vi "EX_1_Llenado tanque máquina de esatados.vi"() -> ()   [LabVIEW 2026]
panel:
  out "MOTOR":bool
  out "V1":bool
  out "V2":bool
  out "VB":bool
  out "TANQUE VB":dbl(slide) scale=0.0..10.0
  out "TANQUE VA":dbl(slide) scale=0.0..10.0
  out "VA":bool
  out "TANQUE 1":dbl(slide) scale=0.0..20.0
  out "TANQUE 2":dbl(slide) scale=0.0..20.0
  in  "Inicio":bool
  in  "DL2":bool
  in  "DL1":bool
  in  "stop":bool
  in  "SP1":bool
  in  "SP2":bool
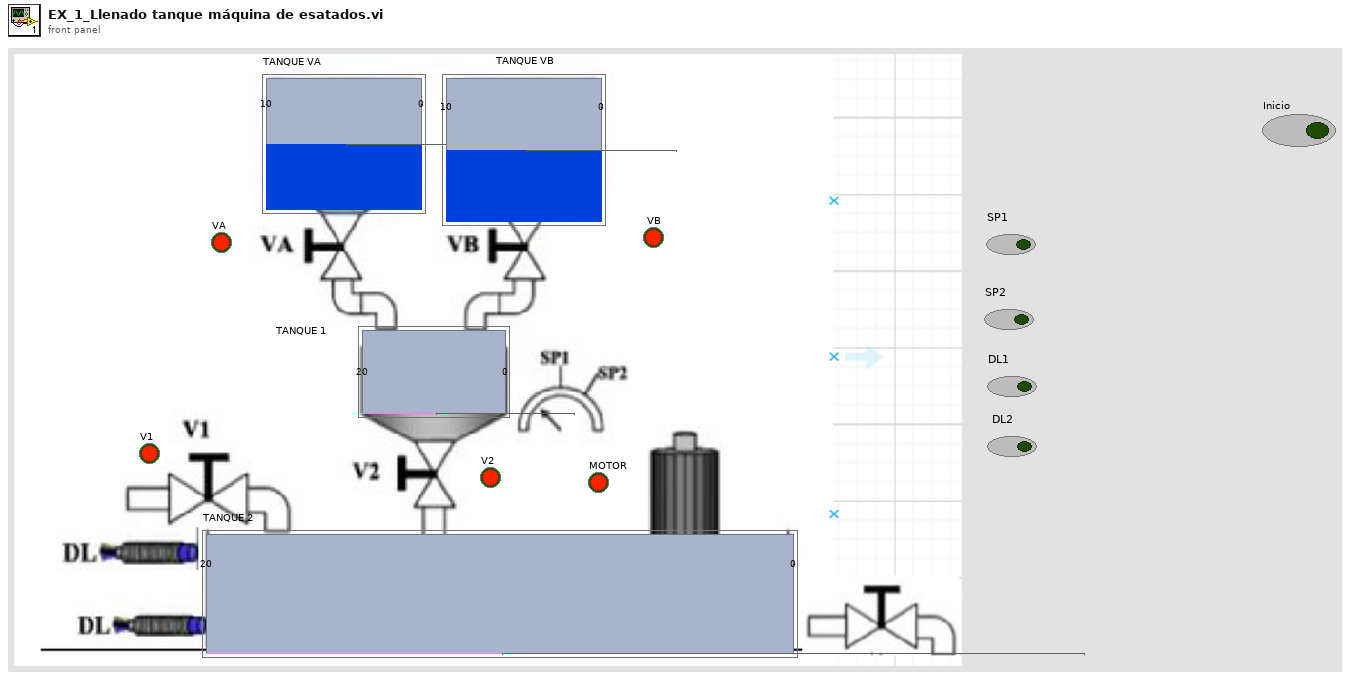
[diagram p1: front panel]
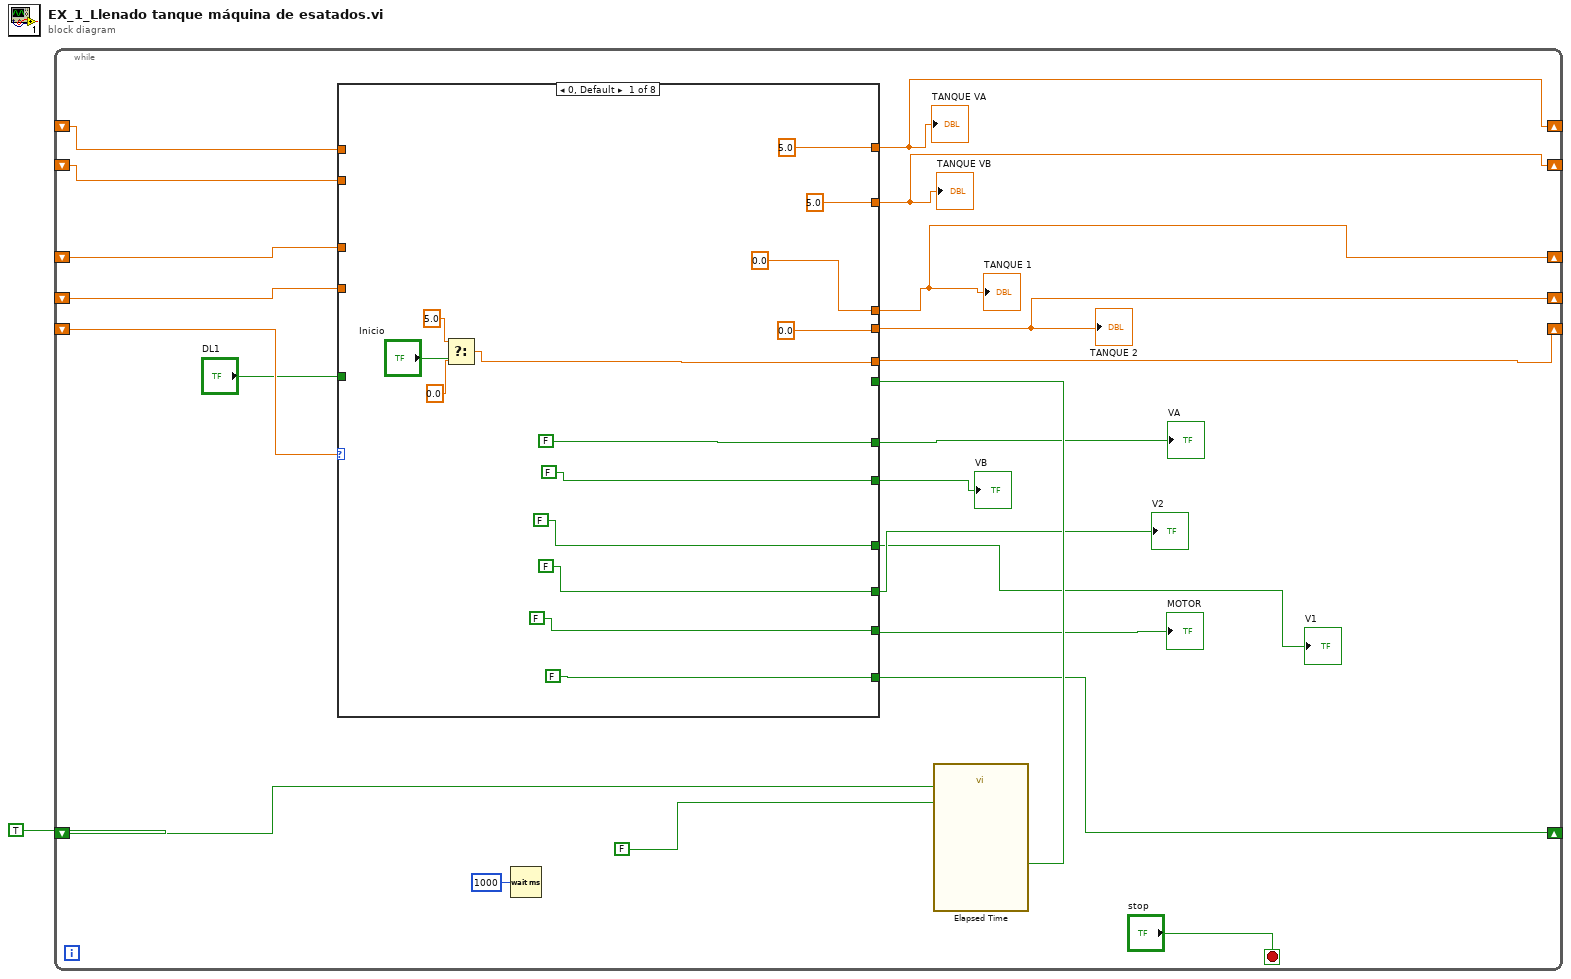
[diagram p0: block diagram]
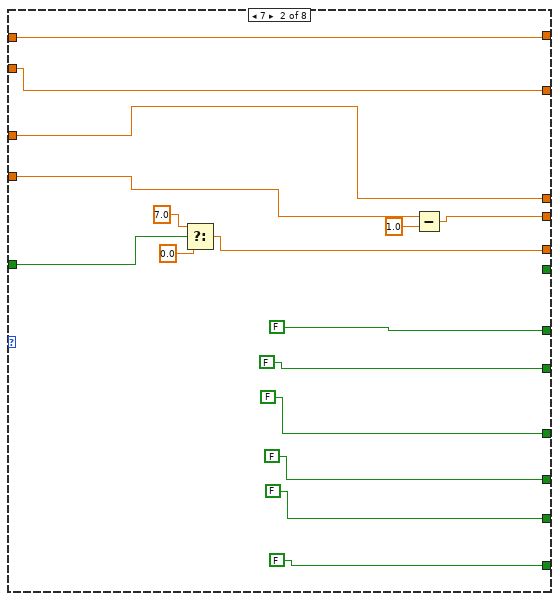
[diagram p2: hidden frame]
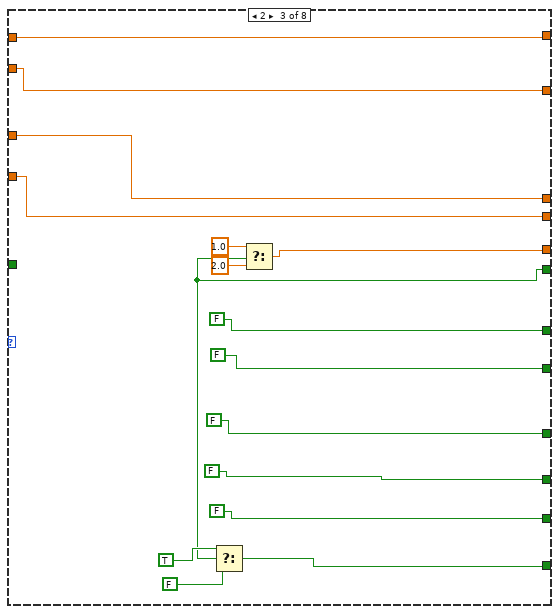
[diagram p3: hidden frame]
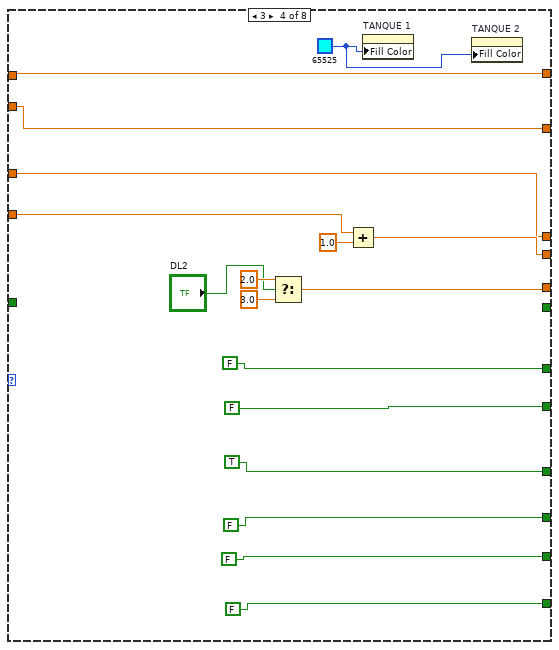
[diagram p4: hidden frame]
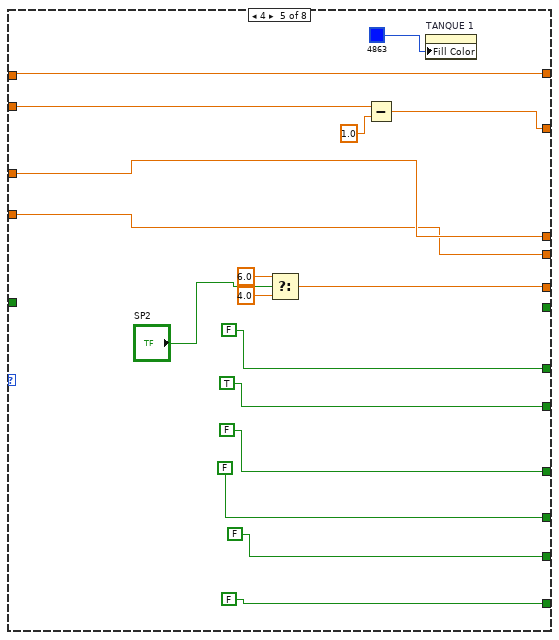
[diagram p5: hidden frame]
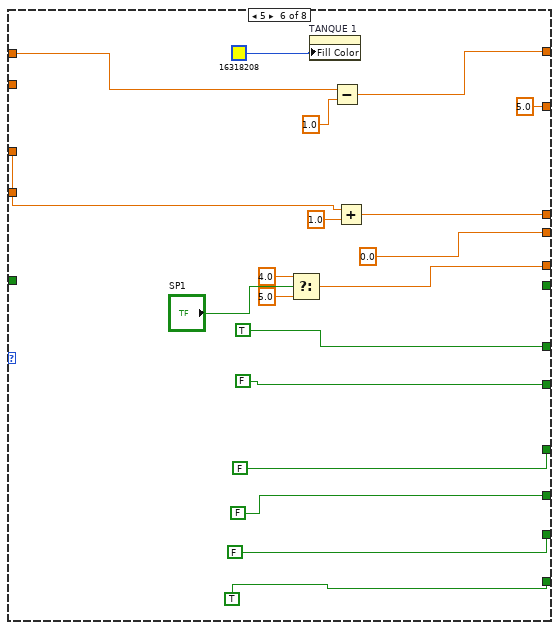
[diagram p6: hidden frame]
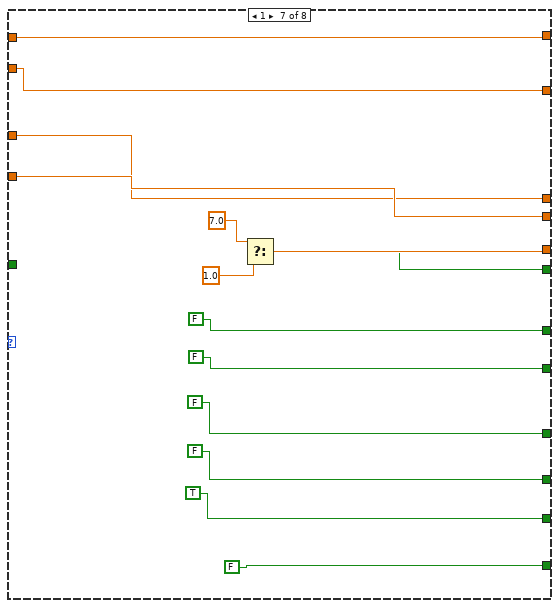
[diagram p7: hidden frame]
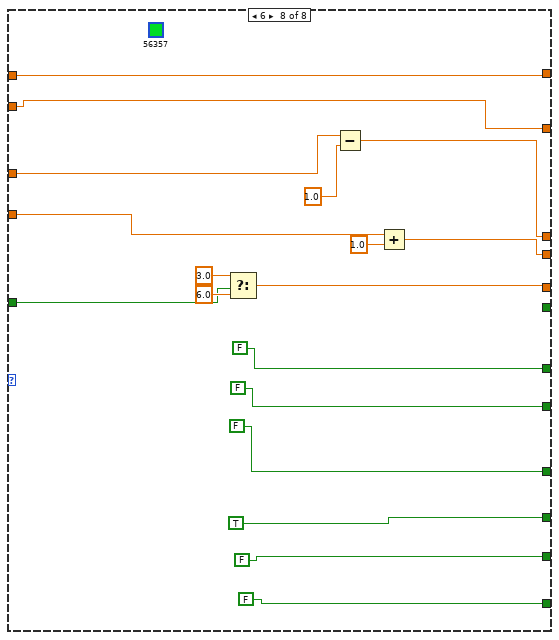
[diagram p8: hidden frame]
diagram:
  n1 = while {
    shift-right: [w21] -> _
    shift-left: _ -> [w23]
    shift-right: [w17] -> _
    shift-left: TRUE -> [w20]
    shift-right: [w13] -> _
    shift-left: _ -> [w14]
    shift-right: [w11] -> _
    shift-left: _ -> [w12]
    shift-right: [w9] -> _
    shift-left: _ -> [w7]
    shift-right: [w8] -> _
    shift-left: _ -> [w5]
    stop <- "stop" stop-if-true
    n2 = Wait (ms)(milliseconds to wait=u32 1000) -> ()  [unwired: 1 out]
    n3 = call "Elapsed Time"("Reset"=w20, "Auto Reset"=FALSE) -> ("Time has Elapsed"=w18:bool)  [unwired: 10 in, 7 out]
    n4 = case shown="0, Default" w23 {
      tunnel: [FALSE FALSE FALSE FALSE FALSE TRUE FALSE FALSE] -> w10
      tunnel: [FALSE FALSE FALSE FALSE TRUE FALSE FALSE FALSE] -> w4
      tunnel: [FALSE FALSE FALSE TRUE FALSE FALSE FALSE FALSE] -> w2
      tunnel: [FALSE FALSE FALSE FALSE FALSE FALSE FALSE TRUE] -> w3
      tunnel: [FALSE FALSE FALSE FALSE FALSE FALSE TRUE FALSE] -> w6
      tunnel: [w30 w53 w64 w81 w96 w116 w129 w150] -> w21
      tunnel: w18 -> [_ _ w58 _ _ _ w128 _]
      tunnel: [FALSE FALSE w59 FALSE FALSE TRUE FALSE FALSE] -> w17
      tunnel: [0.0 w41 w54 w73 w91 0.0 w126 w140] -> w11
      tunnel: "DL1" -> [_ w50 _ _ _ _ _ w145]
      tunnel: w14 -> [_ w40 w57 w72 w93 w109 w125 w144]
      tunnel: [0.0 w40 w57 w72 w93 w108 w125 w139] -> w13
      tunnel: w12 -> [_ w43 w54 w74 w91 _ w126 w142]
      tunnel: [5.0 ("TANQUE VA") w39 w56 w71 w90 w106 w124 w138] -> w9
      tunnel: [5.0 ("TANQUE VB") w38 w55 w70 w89 5.0 ("TANQUE VB") w123 w137] -> w8
      tunnel: w7 -> [_ w39 w56 w71 w90 w107 w124 w138]
      tunnel: w5 -> [_ w38 w55 w70 w88 _ w123 w137]
      frame 0, Default {
        n5 = Select(t=5.0, s="Inicio", f=0.0) -> (s? t:f=w30:dbl)
      }
      frame 7 {
        n6 = Select(t=7.0, s=w50, f=0.0) -> (s? t:f=w53:dbl)
        n7 = Subtract(x=w43, y=1.0) -> (x-y=w41:dbl)
      }
      frame 2 {
        n8 = Select(t=TRUE, s=w58, f=FALSE) -> (s? t:f=w59:bool)
        n9 = Select(t=1.0, s=w58, f=2.0) -> (s? t:f=w64:dbl)
      }
      frame 3 {
        w76 = u32 65525 ("Fill Color")
        n10 = Select(t=2.0, s="DL2", f=3.0) -> (s? t:f=w81:dbl)
        n11 = Add(x=w74, y=1.0) -> (x+y=w73:dbl)
        n12 = property on="TANQUE 1" class="Slide (strict)"("Fill Color"=w76) -> ()  [unwired: 2 in, 2 out]
        n13 = property on="TANQUE 2" class="Slide (strict)"("Fill Color"=w76) -> ()  [unwired: 2 in, 2 out]
      }
      frame 4 {
        n14 = Select(t=6.0, s="SP2", f=4.0) -> (s? t:f=w96:dbl)
        n15 = Subtract(x=w88, y=1.0) -> (x-y=w89:dbl)
        n16 = property on="TANQUE 1" class="Slide (strict)"("Fill Color"=u32 4863) -> ()  [unwired: 2 in, 2 out]
      }
      frame 5 {
        n17 = Select(t=4.0, s="SP1", f=5.0) -> (s? t:f=w116:dbl)
        n18 = property on="TANQUE 1" class="Slide (strict)"("Fill Color"=u32 16318208) -> ()  [unwired: 2 in, 2 out]
        n19 = Subtract(x=w107, y=1.0) -> (x-y=w106:dbl)
        n20 = Add(x=w109, y=1.0) -> (x+y=w108:dbl)
      }
      frame 1 {
        n21 = Select(t=7.0, s=w128, f=1.0) -> (s? t:f=w129:dbl)
      }
      frame 6 {
        (unwired) u32 56357 ("Fill Color")
        n22 = Select(t=3.0, s=w145, f=6.0) -> (s? t:f=w150:dbl)
        n23 = Subtract(x=w144, y=1.0) -> (x-y=w139:dbl)
        n24 = Add(x=w142, y=1.0) -> (x+y=w140:dbl)
      }
    }
    "TANQUE 2" <- w11
    "TANQUE 1" <- w13
    "VA" <- w10
    "VB" <- w4
    "V2" <- w3
    "V1" <- w2
    "MOTOR" <- w6
    "TANQUE VA" <- w9
    "TANQUE VB" <- w8
  }
